vi "CAEN_HVSystem.ProcEvents.vi"(0 "i ref in":refnum<vi>, 5 "error in":errorcluster) -> (14 "i ref out":refnum<vi>, 19 "error out":errorcluster)   [LabVIEW 2014, in "CAEN_HVSystem.lvlib"]
doc: "This method is used to define the events the object will listen to. Add your own events here."
uses:
  CAEN_HVSystem.lvlib
  CSCore/BaseProcess/BaseProcess.event definition.ctl
  CSCore/CAEObj/CAEObj.event definition.ctl
  CSCore/BaseProcess/BaseProcess.descriptor string definition.ctl
  CSCore/BaseProcess/BaseProcess.lvlib
  CSCore/CAEObj/CAEObj.lvlib
panel:
  in  "event definition":T1={"CAEEvtDef"={"URL"="lvmsg://setKill", "enable"=TRUE, "ignoreResID"=FALSE}, "Data Descriptor"="S:1 n[Kill] //If Kill=True: Switch OFF at the max rate all system channels;"}
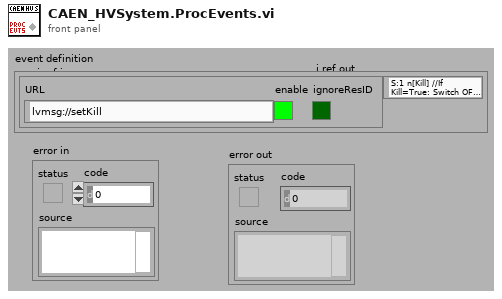
[diagram p1: front panel]
types:
  T1 = typedef "BaseProcess.lvlib/BaseProcess.event definition.ctl" = cluster{"CAEEvtDef":T2, "Data Descriptor":T3}
  T2 = typedef "CAEObj.lvlib/CAEObj.event definition.ctl" = cluster{"URL":string, "enable":bool, "ignoreResID":bool}
  T3 = typedef "BaseProcess.lvlib/BaseProcess.descriptor string definition.ctl" = string
  T4 = typedef "CAEN_HVSystem.lvlib/CAEN_HVSystem.i attribute.ctl" = cluster{"System Name":string, "DIM Service IDs":cluster{"Fan Status":i32}, "SymbolicName":cluster{"SymbolicName":string, "DIM Status":cluster{"no link":bool, "quality":i32, "Time Stamp":timestamp}}, "ModelName":cluster{"ModelName":string, "DIM Status":cluster{"no link":bool, "quality":i32, "Time Stamp":timestamp}}, "Slots":cluster{"Slots":i16, "DIM Status":cluster{"no link":bool, "quality":i32, "Time Stamp":timestamp}}, "Kill":cluster{"Kill":bool, "DIM Status":cluster{"no link":bool, "quality":i32, "Time Stamp":timestamp}}, "ClearAlarm":cluster{"ClearAlarm":bool, "DIM Status":cluster{"no link":bool, "quality":i32, "Time Stamp":timestamp}}, "Sessions":cluster{"Sessions":string, "DIM Status":cluster{"no link":bool, "quality":i32, "Time Stamp":timestamp}}, "SwRelease":cluster{"SwRelease":string, "DIM Status":cluster{"no link":bool, "quality":i32, "Time Stamp":timestamp}}, "GenSignCfg":cluster{"GenSignCfg":i16, "DIM Status":cluster{"no link":bool, "quality":i32, "Time Stamp":timestamp}}, "FrontPanIn":cluster{"FrontPanIn":i16, "DIM Status":cluster{"no link":bool, "quality":i32, "Time Stamp":timestamp}}, "FrontPanOut":cluster{"FrontPanOut":i16, "DIM Status":cluster{"no link":bool, "quality":i32, "Time Stamp":timestamp}}, "HvPwSM":cluster{"HvPwSM":string, "DIM Status":cluster{"no link":bool, "quality":i32, "Time Stamp":timestamp}}, "FanStat":cluster{"FanStat":string, "DIM Status":cluster{"no link":bool, "quality":i32, "Time Stamp":timestamp}}, "ClkFreq":cluster{"ClkFreq":i16, "DIM Status":cluster{"no link":bool, "quality":i32, "Time Stamp":timestamp}}, "HVClkConf":cluster{"HVClkConf":string, "DIM Status":cluster{"no link":bool, "quality":i32, "Time Stamp":timestamp}}, "CnetCrNum":cluster{"CnetCrNum":i16, "DIM Status":cluster{"no link":bool, "quality":i32, "Time Stamp":timestamp}}, "IPAddr":cluster{"IPAddr":string, "DIM Status":cluster{"no link":bool, "quality":i32, "Time Stamp":timestamp}}, "IPNetMsk":cluster{"IPNetMsk":string, "DIM Status":cluster{"no link":bool, "quality":i32, "Time Stamp":timestamp}}, "IPGw":cluster{"IPGw":string, "DIM Status":cluster{"no link":bool, "quality":i32, "Time Stamp":timestamp}}, "RS232Par":cluster{"RS232Par":string, "DIM Status":cluster{"no link":bool, "quality":i32, "Time Stamp":timestamp}}}
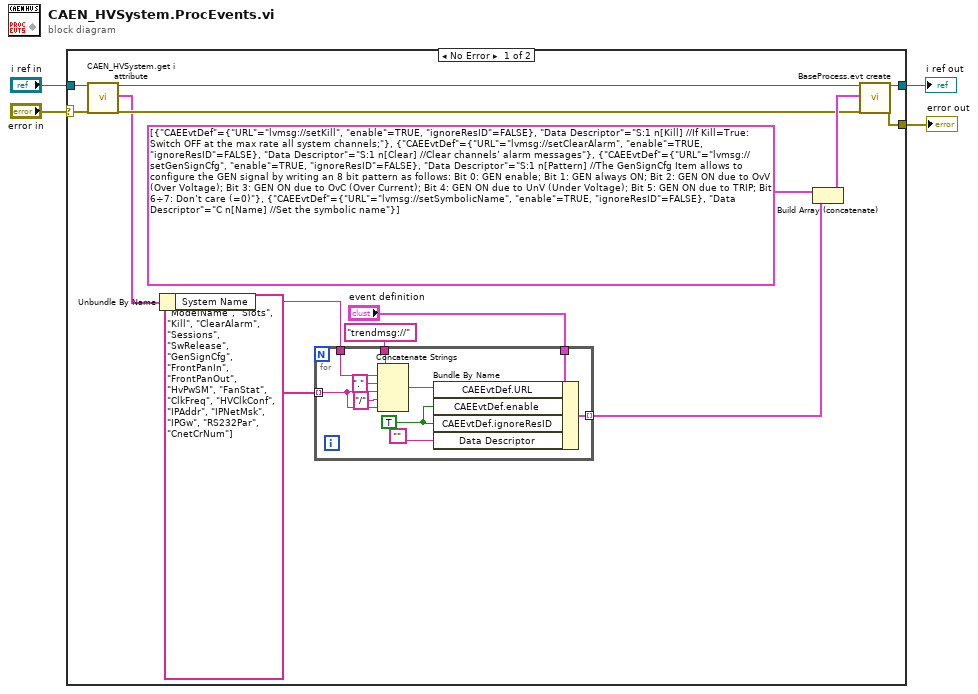
[diagram p0: block diagram]
diagram:
  n1 = case shown="No Error" "error in" {
    selector: "error in" -> [w9 w29]
    tunnel: "i ref in" -> [w10 w30]
    tunnel: [w18 w30] -> w3
    tunnel: [w17 w29] -> w2
    frame No Error {
      n2 = call "CAEN_HVSystem.get i attribute.vi"("i ref in"=w10, "error in (no error)"=w9) -> ("i ref out"=w8:refnum<vi>, "i attribute"=w6:T4, "error out"=w7:errorcluster)  [unwired: 15 in]
      n3 = Unbundle By Name(w6) -> ("System Name"=w5:string)
      n4 = for {
        tunnel: "event definition" -> [w28]
        tunnel: "trendmsg://" -> [w27]
        tunnel: string[] ["SymbolicName", "ModelName", "Slots", "Kill", "ClearAlarm", "Sessions", "SwRelease", "GenSignCfg", "FrontPanIn", "FrontPanOut", "HvPwSM", "FanStat", "ClkFreq", "HVClkConf", "IPAddr", "IPNetMsk", "IPGw", "RS232Par", "CnetCrNum"] -> [w22] mode=indexing
        tunnel: [w21] -> w13 mode=indexing
        tunnel: w5 -> [w20]
        w25 = TRUE ("CAEEvtDef.ignoreResID")
        n5 = Concatenate Strings(w27, w20, "." ("string"), w22, "/" ("string"), w22) -> (w26:string)
        n6 = Bundle By Name(cluster=w28, "CAEEvtDef.URL"=w26, "CAEEvtDef.enable"=w25, "CAEEvtDef.ignoreResID"=w25, "Data Descriptor"="") -> (w21:T1)
      }
      n7 = Build Array (concatenate)(T1[] [{"CAEEvtDef"={"URL"="lvmsg://setKill", "enable"=TRUE, "ignoreResID"=FALSE}, "Data Descriptor"="S:1 n[Kill] //If Kill=True: Switch OFF at the max rate all system channels;"}, {"CAEEvtDef"={"URL"="lvmsg://setClearAlarm", "enable"=TRUE, "ignoreResID"=FALSE}, "Data Descriptor"="S:1 n[Clear] //Clear channels’ alarm messages"}, {"CAEEvtDef"={"URL"="lvmsg://setGenSignCfg", "enable"=TRUE, "ignoreResID"=FALSE}, "Data Descriptor"="S:1 n[Pattern] //The GenSignCfg Item allows to configure the GEN signal by writing an 8 bit pattern as follows: Bit 0: GEN enable; Bit 1: GEN always ON; Bit 2: GEN ON due to OvV (Over Voltage); Bit 3: GEN ON due to OvC (Over Current); Bit 4: GEN ON due to UnV (Under Voltage); Bit 5: GEN ON due to TRIP; Bit 6÷7: Don’t care (=0)"}, {"CAEEvtDef"={"URL"="lvmsg://setSymbolicName", "enable"=TRUE, "ignoreResID"=FALSE}, "Data Descriptor"="C n[Name] //Set the symbolic name"}] ("new events"), w13) -> (w11:T1[])
      n8 = call "BaseProcess.evt create.vi"("i ref in"=w8, "newEvents"=w11, "error in (no error)"=w7) -> ("i ref out"=w18:refnum<vi>, "error out"=w17:errorcluster)  [unwired: 13 in, 2 out]
    }
    frame Error {
    }
  }
  "i ref out" <- w3
  "error out" <- w2
